vi "UpdateRGNArray.vi"(10 "NewROI":T1, 11 "rgn_array in":T2) -> (3 "rgn_array out":T2)   [LabVIEW 2013, in "Photometrics_CH-250_Cam.lvclass"]
uses:
  Photometrics_CH-250_Cam.lvclass
  Point Grey Camera/subVis/ROI_TypDef.ctl
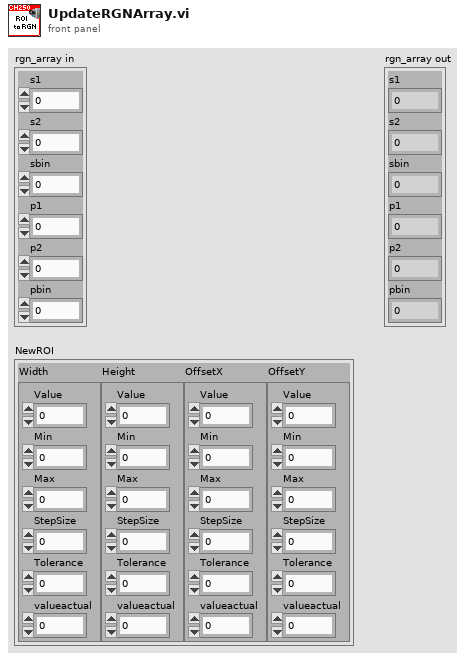
[diagram p1: front panel]
types:
  T1 = typedef "ROI_TypDef.ctl" = cluster{"Width":cluster{"Value":dbl, "Min":dbl, "Max":dbl, "StepSize":dbl, "Tolerance":dbl, "valueactual":dbl}, "Height":cluster{"Value":dbl, "Min":dbl, "Max":dbl, "StepSize":dbl, "Tolerance":dbl, "valueactual":dbl}, "OffsetX":cluster{"Value":dbl, "Min":dbl, "Max":dbl, "StepSize":dbl, "Tolerance":dbl, "valueactual":dbl}, "OffsetY":cluster{"Value":dbl, "Min":dbl, "Max":dbl, "StepSize":dbl, "Tolerance":dbl, "valueactual":dbl}}
  T2 = cluster{"s1":u16, "s2":u16, "sbin":u16, "p1":u16, "p2":u16, "pbin":u16}
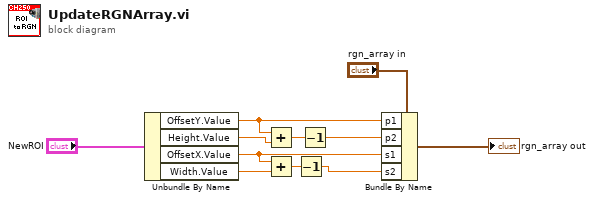
[diagram p0: block diagram]
diagram:
  n1 = Unbundle By Name("NewROI") -> ("OffsetY.Value"=w4:dbl, "Height.Value"=w3:dbl, "OffsetX.Value"=w5:dbl, "Width.Value"=w6:dbl)
  n2 = Add(x=w4, y=w3) -> (x+y=w2:dbl)
  n3 = Add(x=w5, y=w6) -> (x+y=w7:dbl)
  n4 = Decrement(x=w7) -> (x-1=w10:dbl)
  n5 = Decrement(x=w2) -> (x-1=w9:dbl)
  n6 = Bundle By Name(cluster="rgn_array in", "p1"=w4, "p2"=w9, "s1"=w5, "s2"=w10) -> (→"rgn_array out":T2)
